vi "Measurement Launcher.vi"(8 "error in (no error)":errorcluster, 9 "Configuration":variant, 10 "Measurement.UI":refnum<class "Measurement.UI.lvclass">, 11 "Measurement":refnum<class "Measurement.lvclass">) -> (0 "error out":errorcluster)   [LabVIEW 2017]
uses:
  Subsystems/Measurement/Measurement.lvclass
  D:/Program Files (x86)/National Instruments/LabVIEW 2017/vi.lib/JKI/JKI SMO/SMO/SMO.lvclass
  Subsystems/Measurement.UI/Measurement.UI.lvclass
  D:/Program Files (x86)/National Instruments/LabVIEW 2017/vi.lib/JKI/JKI SMO/SMO.UI/SMO.UI.lvclass
  <vilib>/JKI/JKI SMO/SMO/SMO.lvclass
  <vilib>/JKI/JKI SMO/SMO.UI/SMO.UI.lvclass
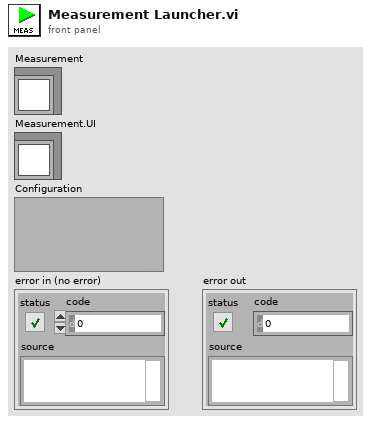
[diagram p1: front panel]
types:
  T1 = typedef "SMO.lvclass/Public Events.ctl" = cluster{"Error":refnum<user-event>, "State":refnum<user-event>, "Reserve State":refnum<user-event>}
  T2 = cluster{"SMO.UI Public Events":refnum<event-registration>, "Event Registration Refnum":refnum<event-registration>, "Measurement Public Events":refnum<event-registration>}
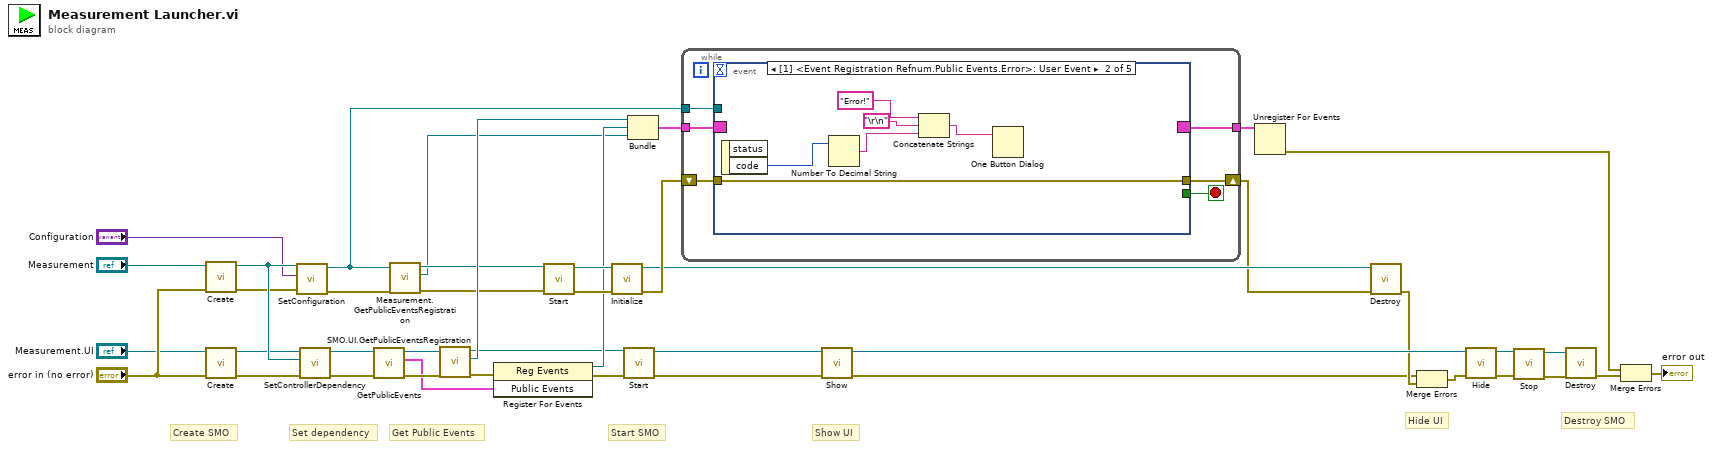
[diagram p0: block diagram]
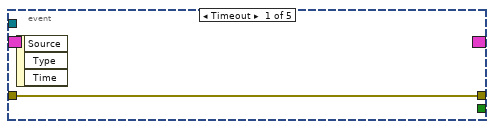
[diagram p2: hidden frame]
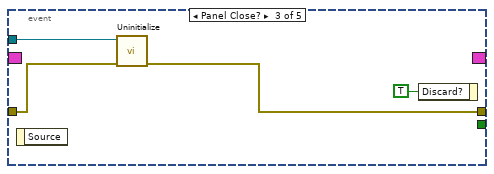
[diagram p3: hidden frame]
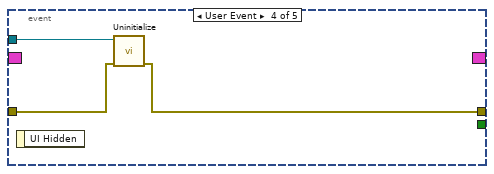
[diagram p4: hidden frame]
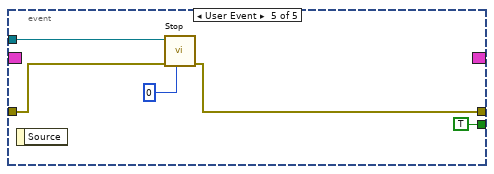
[diagram p5: hidden frame]
diagram:
  # "Set dependency"
  # "Hide UI"
  # "Show UI"
  # "Get Public Events"
  # "Start SMO"
  # "Destroy SMO"
  # "Create SMO"
  n1 = call <vilib>:"Create.vi"("error in (no error)"="error in (no error)", "SMO"="Measurement") -> ("error out"=w17:errorcluster, "SMO out"=w42:refnum<class "Measurement.lvclass">)  [unwired: 7 in, 1 out]
  n2 = call <vilib>:"Create.vi"("error in (no error)"="error in (no error)", "SMO"="Measurement.UI") -> ("error out"=w39:errorcluster, "SMO out"=w38:refnum<class "Measurement.UI.lvclass">)  [unwired: 7 in, 1 out]
  n3 = call "SetConfiguration.vi"("error in (no error)"=w17, "Configuration"="Configuration", "Measurement in"=w42) -> ("error out"=w3:errorcluster, "Measurement out"=w5:refnum<class "Measurement.lvclass">)  [unwired: 7 in]
  n4 = call "SetControllerDependency.vi"("error in (no error)"=w39, "Measurement"=w42, "Measurement.UI in"=w38) -> ("error out"=w40:errorcluster, "Measurement.UI out"=w41:refnum<class "Measurement.UI.lvclass">)  [unwired: 7 in]
  n5 = call <vilib>:"GetPublicEvents.vi"("error in (no error)"=w40, "SMO"=w41) -> ("error out"=w29:errorcluster, "Public Events"=w16:T1, "SMO out"=w28:refnum<class "Measurement.UI.lvclass">)  [unwired: 7 in]
  n6 = call "Measurement.GetPublicEventsRegistration.vi"("error in (no error)"=w3, "Measurement in"=w5) -> ("error out"=w2:errorcluster, "Measurement Public Events"=w1:refnum<event-registration>, "Measurement out"=w4:refnum<class "Measurement.lvclass">)  [unwired: 7 in]
  n7 = call <vilib>:"SMO.UI.GetPublicEventsRegistration.vi"("error in (no error)"=w29, "SMO.UI"=w28) -> ("error out"=w31:errorcluster, "SMO.UI Public Events"=w33:refnum<event-registration>, "SMO.UI out"=w30:refnum<class "Measurement.UI.lvclass">)  [unwired: 7 in]
  n8 = register-events(error in=w31, w16) -> (reference out=w32:refnum<event-registration>, error out=w15:errorcluster)  [unwired: 1 in]
  n9 = call <vilib>:"Start.vi"("error in (no error)"=w2, "SMO"=w4) -> ("error out"=w35:errorcluster, "SMO out"=w34:refnum<class "Measurement.lvclass">)  [unwired: 8 in]
  n10 = call "Initialize.vi"("error in (no error)"=w35, "Measurement in"=w34) -> ("error out"=w36:errorcluster, "Measurement out"=w7:refnum<class "Measurement.lvclass">)  [unwired: 8 in]
  n11 = call <vilib>:"Start.vi"("error in (no error)"=w15, "SMO"=w30) -> ("error out"=w13:errorcluster, "SMO out"=w12:refnum<class "Measurement.UI.lvclass">)  [unwired: 8 in]
  n12 = Bundle("SMO.UI Public Events"=w33, "Event Registration Refnum"=w32, "Measurement Public Events"=w1) -> (w18:T2)  [unwired: 1 in]
  n13 = while {
    shift-right: [w48] -> w6
    shift-left: w36 -> [w47]
    tunnel: w18 -> [w44]
    tunnel: [w46] -> w19
    tunnel: w5 -> [w45]
    stop <- w49 stop-if-true
    n14 = event shown="[1] <Event Registration Refnum.Public Events.Error>: User Event" {
      selector: w44 -> [_ _ _ _ _]
      dyn-events: [_ _ _ _ _] -> w46
      timeout: _ -> [_ _ _ _ _]
      tunnel: [_ _ _ _ TRUE ("OK")] -> w49
      tunnel: w45 -> [_ _ w59 w63 w67]
      tunnel: [w50 w56 w57 w61 w64] -> w48
      tunnel: w47 -> [w50 w56 w58 w62 w65]
      event Timeout {
        n15 = event-data() -> ()  [unwired: 1 in, 3 out]
      }
      event User Event {
        n16 = event-data() -> ("code"=w55:i32)  [unwired: 1 in, 1 out]
        n17 = Number To Decimal String(number=w55) -> (decimal integer string=w52:string)  [unwired: 1 in]
        n18 = Concatenate Strings("Error!" ("string"), "\r\n", w52) -> (w53:string)
        n19 = One Button Dialog(message=w53) -> ()  [unwired: 1 in, 1 out]
      }
      event Panel Close? {
        n20 = event-data() -> ()  [unwired: 1 in, 1 out]
        n21 = call "Uninitialize.vi"("error in (no error)"=w58, "Measurement in"=w59) -> ("error out"=w57:errorcluster)  [unwired: 8 in, 1 out]
        n22 = event-data("Discard?"=TRUE ("OK")) -> ()  [unwired: 1 in, 1 out]
      }
      event User Event {
        n23 = event-data() -> ()  [unwired: 1 in, 1 out]
        n24 = call "Uninitialize.vi"("error in (no error)"=w62, "Measurement in"=w63) -> ("error out"=w61:errorcluster)  [unwired: 8 in, 1 out]
      }
      event User Event {
        n25 = event-data() -> ()  [unwired: 1 in, 1 out]
        n26 = call <vilib>:"Stop.vi"("timeout in ms (-1)"=0, "error in (no error)"=w65, "SMO"=w67) -> ("error out"=w64:errorcluster)  [unwired: 7 in, 1 out]
      }
    }
  }
  n27 = call <vilib>:"Show.vi"("error in (no error)"=w13, "SMO.UI"=w12) -> ("error out"=w14:errorcluster, "SMO.UI out"=w21:refnum<class "Measurement.UI.lvclass">)  [unwired: 8 in]
  n28 = Unregister For Events(event registration refnum=w19) -> (error out=w10:errorcluster)  [unwired: 1 in]
  n29 = call <vilib>:"Destroy.vi"("error in (no error)"=w6, "SMO"=w7) -> ("error out"=w20:errorcluster)  [unwired: 9 in]
  n30 = Merge Errors(w14, w20) -> (w22:errorcluster)
  n31 = call <vilib>:"Hide.vi"("error in (no error)"=w22, "SMO.UI"=w21) -> ("error out"=w24:errorcluster, "SMO.UI out"=w23:refnum<class "Measurement.UI.lvclass">)  [unwired: 8 in]
  n32 = call <vilib>:"Stop.vi"("error in (no error)"=w24, "SMO"=w23) -> ("error out"=w25:errorcluster, "SMO out"=w26:refnum<class "Measurement.UI.lvclass">)  [unwired: 8 in]
  n33 = call <vilib>:"Destroy.vi"("error in (no error)"=w25, "SMO"=w26) -> ("error out"=w11:errorcluster)  [unwired: 9 in]
  n34 = Merge Errors(w10, w11) -> (→"error out":errorcluster)
